vi "NIIE_Move.vi"(8 "Error":errorcluster, 9 "Point(x,y)":cluster{"x":i16, "y":i16}, 10 "Tools":T8=enum."Ellipse", 11 "Data":T1={"Class"={"Ants"=refnum, "Layer"=refnum, "Templates"=refnum, "Icon"=refnum, "Glyph"=refnum, "Settings"=refnum, "Tools"=refnum}, "Ref"={"Add Layer"=refnum, "Remove Layer"=refnum, "Line Text"=[], "Body Text Spec"=refnum, "DNL_Font"=refnum, "glyph path str"=refnum, "templates path str"=refnum, "Arrow Up"=refnum, "Arrow Down"=refnum, "IE VI Ref"=refnum, "Glyphs tree"=refnum, "Templates tree"=refnum, "Layer Icon Text"=refnum, "Layer Template"=refnum, "Clipboard"=refnum, "BW icon in"=refnum, "Color icon in"=refnum, "Layer Clust"=refnum, "Body Text"=refnum, "DNL_Framework Templates"=refnum, "Search Templates"=refnum, "TextMarker"=refnum, "Tab Control"=refnum, "Search Glyphs"=refnum, "Line Color"=refnum, "DNL_Glyphs []"=refnum, "Fill Color"=refnum, "Tools"=refnum, "Glyphs tree"=refnum, "Icon"=refnum, "Preview"=refnum, "Ants"=refnum, "Terminals"=refnum, "menu reference"=refnum, "LayerNames"=[], "GlyphLoadAnimation"=refnum, "TemplateLoadAnimation"=refnum, "refreshGlyphs"=refnum, "refreshTemplates"=refnum}, "Support"={"AntsRect"={"left"=0, "top"=0, "right"=0, "bottom"=0}, "Mouse Move Coords"={"Horizontal"=0, "Vertical"=0}, "Mouse Down Coords"={"Horizontal"=0, "Vertical"=0}, "Temp Coord"={"Horizontal"=0, "Vertical"=0}, "Action"=enum."Default", "Edge Color"=4914962, "Fill Color"=16860, "Mouse Down?"=FALSE, "Draft Mode?"=FALSE, "Temp Icon"=bytes[3102], "CTRL Pressed"=FALSE, "Move Selection?"=FALSE, "AntsRect Orig"={"left"=0, "top"=0, "right"=0, "bottom"=0}, "Text"="", "TM Set?"=FALSE, "Mouse inside icon?"=FALSE, "Tool (old value)"=0, "Pencil Move Color"=0, "Swap Colors?"=FALSE, "Shift pressed?"=FALSE}}) -> (0 "Error Out":errorcluster, 1 "Origin Out":T5, 2 "Active Layer Out":i32, 3 "Data Out":T1={"Class"={"Ants"=refnum, "Layer"=refnum, "Templates"=refnum, "Icon"=refnum, "Glyph"=refnum, "Settings"=refnum, "Tools"=refnum}, "Ref"={"Add Layer"=refnum, "Remove Layer"=refnum, "Line Text"=[], "Body Text Spec"=refnum, "DNL_Font"=refnum, "glyph path str"=refnum, "templates path str"=refnum, "Arrow Up"=refnum, "Arrow Down"=refnum, "IE VI Ref"=refnum, "Glyphs tree"=refnum, "Templates tree"=refnum, "Layer Icon Text"=refnum, "Layer Template"=refnum, "Clipboard"=refnum, "BW icon in"=refnum, "Color icon in"=refnum, "Layer Clust"=refnum, "Body Text"=refnum, "DNL_Framework Templates"=refnum, "Search Templates"=refnum, "TextMarker"=refnum, "Tab Control"=refnum, "Search Glyphs"=refnum, "Line Color"=refnum, "DNL_Glyphs []"=refnum, "Fill Color"=refnum, "Tools"=refnum, "Glyphs tree"=refnum, "Icon"=refnum, "Preview"=refnum, "Ants"=refnum, "Terminals"=refnum, "menu reference"=refnum, "LayerNames"=[], "GlyphLoadAnimation"=refnum, "TemplateLoadAnimation"=refnum, "refreshGlyphs"=refnum, "refreshTemplates"=refnum}, "Support"={"AntsRect"={"left"=0, "top"=0, "right"=0, "bottom"=0}, "Mouse Move Coords"={"Horizontal"=0, "Vertical"=0}, "Mouse Down Coords"={"Horizontal"=0, "Vertical"=0}, "Temp Coord"={"Horizontal"=0, "Vertical"=0}, "Action"=enum."Default", "Edge Color"=4914962, "Fill Color"=16860, "Mouse Down?"=FALSE, "Draft Mode?"=FALSE, "Temp Icon"=bytes[3102], "CTRL Pressed"=FALSE, "Move Selection?"=FALSE, "AntsRect Orig"={"left"=0, "top"=0, "right"=0, "bottom"=0}, "Text"="", "TM Set?"=FALSE, "Mouse inside icon?"=FALSE, "Tool (old value)"=0, "Pencil Move Color"=0, "Swap Colors?"=FALSE, "Shift pressed?"=FALSE}})   [LabVIEW 2021]
uses:
  MB CORE/TypeDefs/Cluster_Button Draw Tools.ctl
  MB CORE/TypeDefs/Bool_Draw Tool.ctl
  MB CORE/TypeDefs/Bool_Line Tool.ctl
  MB CORE/TypeDefs/Bool_ColorExtractor Tool.ctl
  MB CORE/TypeDefs/Bool_Fill Tool.ctl
  MB CORE/TypeDefs/Bool_IERect Tool.ctl
  MB CORE/TypeDefs/Bool_FRect Tool.ctl
  MB CORE/TypeDefs/Bool_Circle Tool.ctl
  MB CORE/TypeDefs/Bool_FillCircle Tool.ctl
  MB CORE/TypeDefs/Bool_Eraser Tool.ctl
  MB CORE/TypeDefs/Bool_Text Tool.ctl
  MB CORE/TypeDefs/Bool_Selection Tool.ctl
  MB CORE/TypeDefs/Bool_Move Tool.ctl
  <vilib>/Utility/miscctls.llb/LVPoint32TypeDef.ctl
  Controls/IE Data.ctl
  Class/Ants/Ants.lvclass
  Class/FakedArray/FakedArray.lvclass
  vi.lib/LabVIEW Icon API/lv_icon/Classes/Icon/Icon.lvclass
  Class/Icon Library/Glyph.lvclass
  Class/Settings/Settings.lvclass
  Class/Tools/Tools Paint.lvclass
  Controls/IE Classes.ctl
  Controls/References Cluster.ctl
  Controls/SupportClass.ctl
  Controls/ENUM_SupportClass_Action.ctl
  vi.lib/LabVIEW Icon API/lv_icon/Controls/IEColor.ctl
  vi.lib/LabVIEW Icon API/lv_icon/Classes/Layer/Layer.lvclass
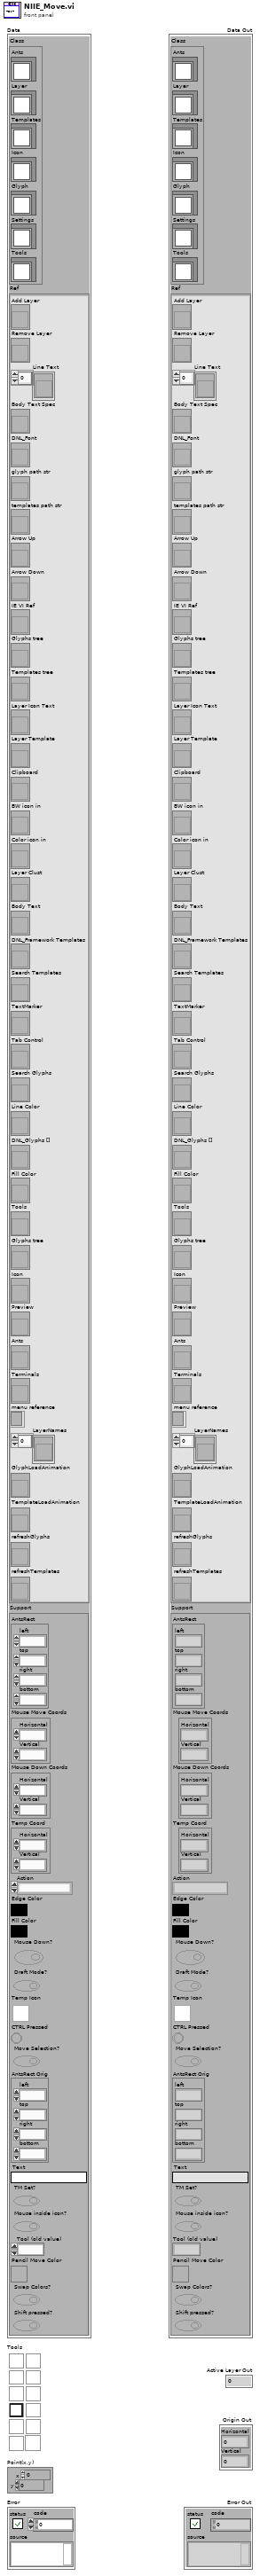
[diagram p1: front panel]
types:
  T1 = typedef "IE Data.ctl" = cluster{"Class":T2, "Ref":T3, "Support":T4}
  T2 = typedef "IE Classes.ctl" = cluster{"Ants":refnum<class "Ants.lvclass">, "Layer":refnum<class "FakedArray.lvclass">, "Templates":refnum<class "FakedArray.lvclass">, "Icon":refnum<class "Icon.lvclass">, "Glyph":refnum<class "Glyph.lvclass">, "Settings":refnum<class "Settings.lvclass">, "Tools":refnum<class "Tools Paint.lvclass">}
  T3 = typedef "References Cluster.ctl" = cluster{"Add Layer":refnum<vi>, "Remove Layer":refnum<vi>, "Line Text":refnum<vi>[], "Body Text Spec":refnum<vi>, "DNL_Font":refnum<vi>, "glyph path str":refnum<vi>, "templates path str":refnum<vi>, "Arrow Up":refnum<vi>, "Arrow Down":refnum<vi>, "IE VI Ref":refnum<vi>, "Glyphs tree":refnum<vi>, "Templates tree":refnum<vi>, "Layer Icon Text":refnum<vi>, "Layer Template":refnum<vi>, "Clipboard":refnum<vi>, "BW icon in":refnum<vi>, "Color icon in":refnum<vi>, "Layer Clust":refnum<vi>, "Body Text":refnum<vi>, "DNL_Framework Templates":refnum<vi>, "Search Templates":refnum<vi>, "TextMarker":refnum<vi>, "Tab Control":refnum<vi>, "Search Glyphs":refnum<vi>, "Line Color":refnum<vi>, "DNL_Glyphs []":refnum<vi>, "Fill Color":refnum<vi>, "Tools":refnum<vi>, "Glyphs tree":refnum<vi>, "Icon":refnum<vi>, "Preview":refnum<vi>, "Ants":refnum<vi>, "Terminals":refnum<vi>, "menu reference":refnum<k9>, "LayerNames":refnum<vi>[], "GlyphLoadAnimation":refnum<vi>, "TemplateLoadAnimation":refnum<vi>, "refreshGlyphs":refnum<vi>, "refreshTemplates":refnum<vi>}
  T4 = typedef "SupportClass.ctl" = cluster{"AntsRect":cluster{"left":i16, "top":i16, "right":i16, "bottom":i16}, "Mouse Move Coords":T5, "Mouse Down Coords":T5, "Temp Coord":T5, "Action":T6, "Edge Color":T7, "Fill Color":T7, "Mouse Down?":bool, "Draft Mode?":bool, "Temp Icon":picture, "CTRL Pressed":bool, "Move Selection?":bool, "AntsRect Orig":cluster{"left":i16, "top":i16, "right":i16, "bottom":i16}, "Text":string, "TM Set?":bool, "Mouse inside icon?":bool, "Tool (old value)":u32, "Pencil Move Color":u32, "Swap Colors?":bool, "Shift pressed?":bool}
  T5 = typedef "LVPoint32TypeDef.ctl" = cluster{"Horizontal":i32, "Vertical":i32}
  T6 = typedef "ENUM_SupportClass_Action.ctl" = enum16{"Default", "Move Selection", "Glyph Library", "Tool"}
  T7 = typedef "IEColor.ctl" = u32
  T8 = typedef "Cluster_Button Draw Tools.ctl" = enum32{"Pencil", "Line", "Dropper", "Fill", "Rectangle", "Filled Rectangle", "Ellipse", "Filled Ellipse", "Eraser", "Text", "Select", "Move"}
  T9 = typedef "LVPositionTypeDef.ctl" = cluster{"Left":i32, "Top":i32}
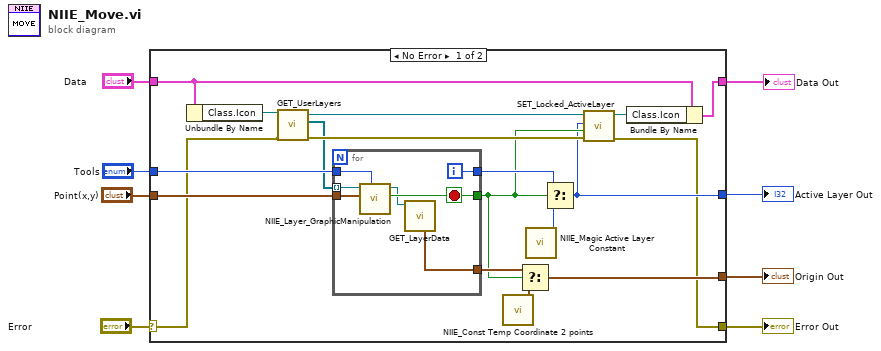
[diagram p0: block diagram]
diagram:
  n1 = case shown="No Error" "Error" {
    selector: "Error" -> [w13 w35]
    tunnel: [w9 w35] -> w7
    tunnel: "Tools" -> [w26 _]
    tunnel: "Point(x,y)" -> [w25 _]
    tunnel: [w16 _] -> w4
    tunnel: [w24 _] -> w3
    tunnel: "Data" -> [w12 w34]
    tunnel: [w10 w34] -> w1
    frame No Error {
      n2 = Unbundle By Name(w12) -> ("Class.Icon"=w14:refnum<class "Icon.lvclass">)
      n3 = call-dynamic "GET_UserLayers.vi"("error in (no error)"=w13, "Icon.lvclass in"=w14) -> ("error out"=w21:errorcluster, "All Layers"=w18:refnum<class "Layer.lvclass">[], "Icon.lvclass out"=w22:refnum<class "Icon.lvclass">)  [unwired: 7 out]
      n4 = for {
        tunnel: w26 -> [w33]
        tunnel: w25 -> [w32]
        tunnel: w18 -> [w31] mode=indexing
        tunnel: [w30] -> w17
        tunnel: [w29] -> w23
        tunnel: [w27] -> w20
        i -> [w29]
        stop <- w30 stop-if-true
        n5 = call "NIIE_Layer_GraphicManipulation.vi"("Radio Buttons"=w33, "Position"=w32, "Layer.lvclass"=w31) -> ("Operation Processed? Out"=w30:bool, "Layer.lvclass Out"=w28:refnum<class "Layer.lvclass">)  [unwired: 1 in, 6 out]
        n6 = call-dynamic "GET_LayerData.vi"("Layer.lvclass in"=w28) -> ("Origin"=w27:T9)  [unwired: 1 in, 9 out]
      }
      n7 = call "NIIE_Const Temp Coordinate 2 points.vi"() -> ("Const Temp Coordinate"=w19:T5)  [unwired: 11 out]
      n8 = Select(t=w20, s=w17, f=w19) -> (s? t:f=w24:T5)
      n9 = call "NIIE_Magic Active Layer Constant.vi"() -> ("Magic Constant"=w15:i32)  [unwired: 11 in]
      n10 = Select(t=w23, s=w17, f=w15) -> (s? t:f=w16:i32)
      n11 = call-dynamic "SET_Locked_ActiveLayer.vi"("error in (no error)"=w21, "Layers Locked?"=w17, "Active Layer"=w16, "Icon.lvclass in"=w22) -> ("error out"=w9:errorcluster, "Icon.lvclass out"=w11:refnum<class "Icon.lvclass">)  [unwired: 6 out]
      n12 = Bundle By Name(cluster=w12, "Class.Icon"=w11) -> (w10:T1)
    }
    frame Error {
    }
  }
  "Error Out" <- w7
  "Active Layer Out" <- w4
  "Origin Out" <- w3
  "Data Out" <- w1
